vi "Update System State.vi"(8 "error in":errorcluster, 11 "Fault Handler in":refnum<class "Fault Handler.lvclass">) -> (0 "error out":errorcluster, 3 "Fault Handler out":refnum<class "Fault Handler.lvclass">)   [LabVIEW 2023, in "Fault Handler.lvlib" / "Fault Handler.lvclass"]
doc: "This routine inspects the state data and transmits an update state command to transition from no fault, or active fault states to a warning, error, or the previous state."
uses:
  Library/Fault Handler.lvclass
  Library/Fault Handler.lvclass/Fault Handler.ctl
  Accessors/Read Error State.vi
  builds/Engine/Engine.lvlibp/Project/Engine.lvclass
  C:/Users/Public/Documents/Development/builds/Engine/Engine.lvlibp/Project/Engine.lvclass
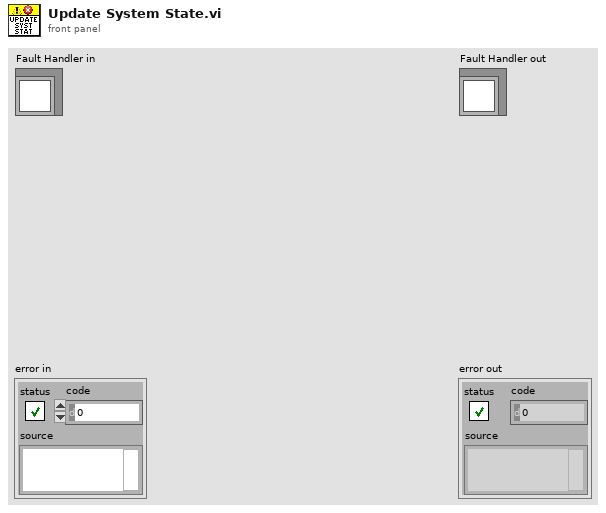
[diagram p1: front panel]
types:
  T1 = typedef "Engine.lvlibp/Engine.lvclass/System Status.ctl" = enum16{"Logged Off", "UUT_Info_Missing", "Idle", "Error", "Warning", "Loading", "Config", "Manual", "Automation", "Report_View", "Previous"}
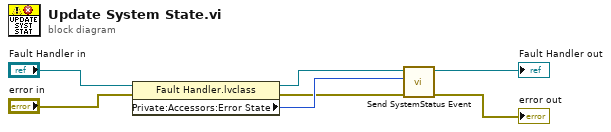
[diagram p0: block diagram]
diagram:
  n1 = property class="Fault Handler.lvclass"(reference="Fault Handler in", error in="error in") -> (reference out=w5:refnum<class "Fault Handler.lvclass">, error out=w3:errorcluster, "Private:Accessors:Error State"=w4:T1)
  n2 = call "Send SystemStatus Event.vi"("error in"=w3, "SystemStatus"=w4, "Engine in"=w5) -> ("error out"=→"error out":errorcluster, "Engine out"=→"Fault Handler out":refnum<class "Fault Handler.lvclass">)  [unwired: 7 in]
